vi "TEST-JSON-RPC+caraya.vi"(8 "error in (no error)":errorcluster) -> (0 "error out":errorcluster)   [LabVIEW 2019]
uses:
  TEST-JSON-RPC--Cluster.ctl
  <vilib>/numeric/Random Number (Range) DBL.vi
  <vilib>/numeric/Random Number (Range) I64.vi
  423c0946-e876-4033-917c-c4e0f5a656b4.vi
  545e0fdc-708c-4040-a6f5-a4d862a94354.vi
  85357fc9-3c23-47d6-a25c-dbb7056a88c4.vi
  9d79f0c2-35ce-467d-8164-7d449b6aa026.vi
  53d3177d-6787-4563-b3f2-ec7d47ca270a.vi
  d9266a12-4538-4804-ad7c-12d0542650b7.vi
  f59088ab-3144-40f5-84fa-71997c4bd8c3.vi
  <vilib>/numeric/sub_Random U32.vi
  <vilib>/JDP Science/JSONtext/JSON text to Variant (path).vi
  <vilib>/JDP Science/JSONtext/Find Item.vi
  <vilib>/JDP Science/JSONtext/Next JSON Value.vi
  <vilib>/JDP Science/JSONtext/String Subset.vi
  <vilib>/JDP Science/JSONtext/Parsing/Advance past next JSON Value (inlined COPY).vi
  <vilib>/JDP Science/JSONtext/Parsing/Advance past whitespace.vi
  <vilib>/JDP Science/JSONtext/Parsing/Advance past String.vi
  <vilib>/JDP Science/JSONtext/Parsing/Advance past Number.vi
  <vilib>/JDP Science/JSONtext/Parsing/Advance past Line Ending.vi
  <vilib>/JDP Science/JSONtext/JSON text to Variant.vi
  <vilib>/Utility/Data Type/Get Type Information.vi
  <vilib>/JDP Science/JSONtext/Parsing/Parse Full Path or Item Name.vi
  <vilib>/JDP Science/JSONtext/Parsing/Advance past Array.vi
  <vilib>/JDP Science/JSONtext/Parsing/Advance past Object.vi
  <vilib>/JDP Science/JSONtext/support/Error Cluster From Code.vi
  <vilib>/JDP Science/JSONtext/Offset/Find Item Locations by Path.vi
  <vilib>/addons/_JKI Toolkits/Caraya/classes/Assert/Assert Almost Equal_Float.vi
  <vilib>/JDP Science/JSONtext/LVClass Serializer/JSONtext LVClass Serializer.lvclass
  JSON-RPC/JSON-RPC.lvclass
  <vilib>/JDP Science/JSONtext/JSONtext.lvlib
  <vilib>/addons/_JKI Toolkits/Caraya/classes/Test/Test.lvclass
  <vilib>/addons/_JKI Toolkits/Caraya/classes/Assert/Assert.lvclass
  <vilib>/Utility/Data Type/NI_Data Type.lvlib
panel:
  out "Elements":dbl[](array[numeric])
  out "Names 3":string[](array[string])
  out "Params 3":string[](array[string])
  out "Array 2":dbl[][](array[numeric])
  out "Array":T1[](array[typedef])
  out "Clusters Section":dbl[](array[numeric])
  out "Arrays":dbl[][](array[numeric])
  out "Clusters":T1[](array[typedef])
  out "Params 2":string[](array[string])
  out "Names 2":string[](array[string])
  out "Params":string[](array[string])
  out "Names":string[](array[string])
  out "REQ.Methods":string
  out "Match?":bool
  out "{JSON} Response":string
  out "{JSON} Requests":string
  out "4. parse response":dbl format="%#_6p"
  out "3. create response":dbl format="%#_6p"
  out "2. parse request":dbl format="%#_6p"
  out "1. create request":dbl format="%#_6p"
  out "REQ.Params":string
  out "results":string
  in  "Numeric":i32=3
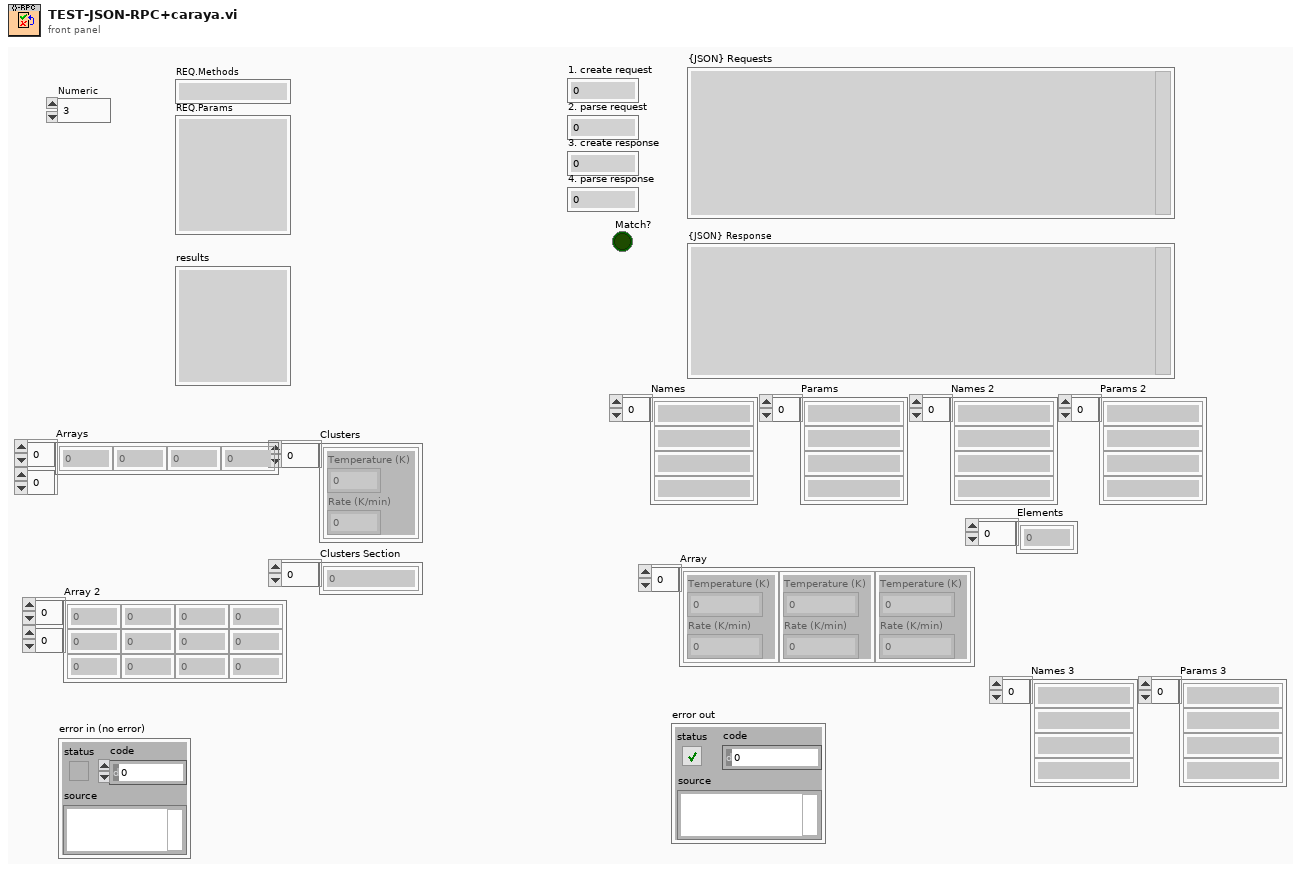
[diagram p1: front panel]
types:
  T1 = typedef "TEST-JSON-RPC--Cluster.ctl" = cluster{"Temperature (K)":dbl, "Rate (K/min)":dbl}
  T2 = enum16{"Parse Error", "Invalid Request", "Method not found", "Invalid params", "Internal error", "Server error"}
  T3 = cluster{"Temperature (K)":dbl, "Rate (K/min)":dbl}
  T4 = typedef "JSONtext.lvlib/JSON Value Type.ctl" = enum16{"Not a JSON Value", "JSON Object", "JSON Array", "String", "Number", "true", "false", "null"}
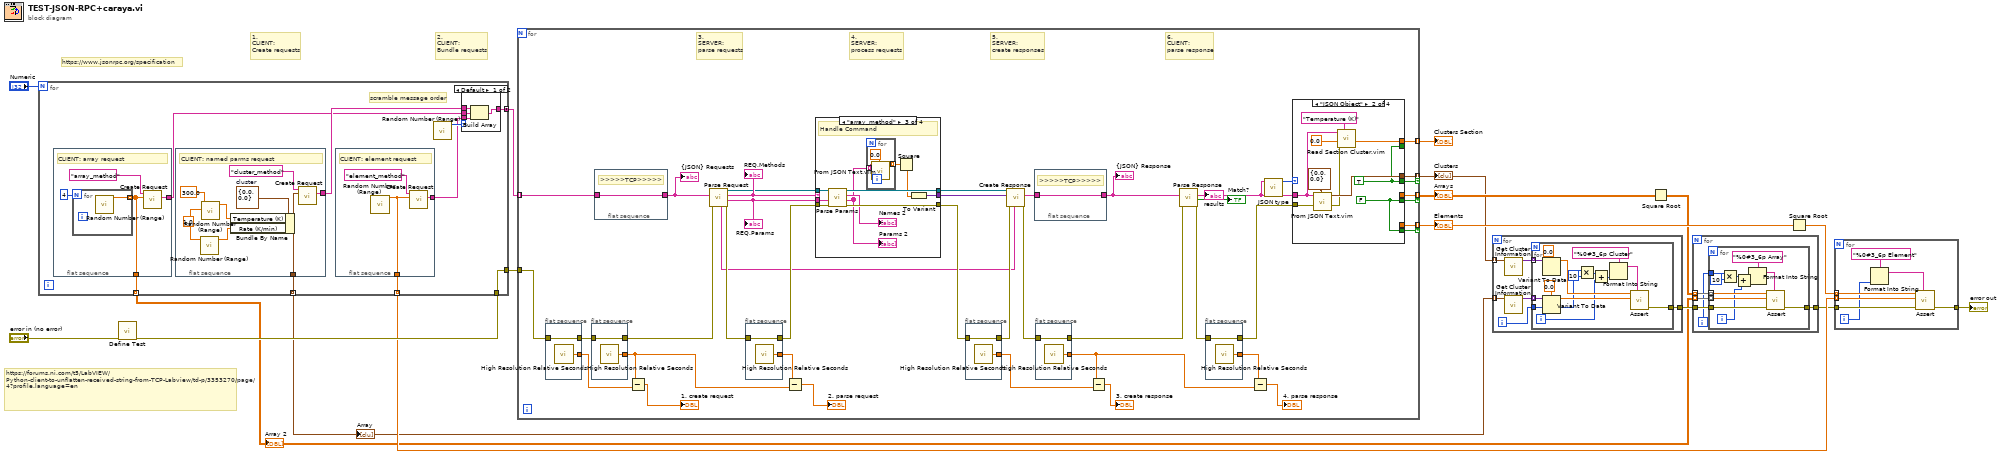
[diagram p0: block diagram]
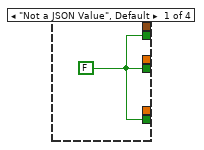
[diagram p2: hidden frame]
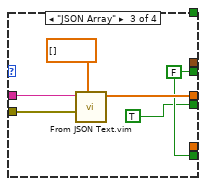
[diagram p3: hidden frame]
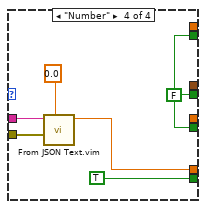
[diagram p4: hidden frame]
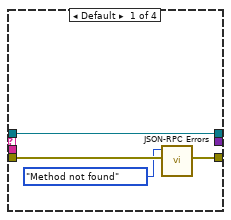
[diagram p5: hidden frame]
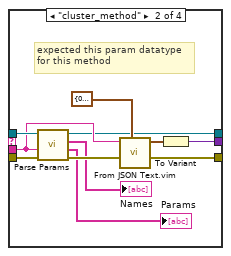
[diagram p6: hidden frame]
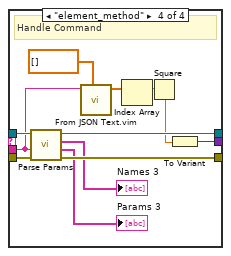
[diagram p7: hidden frame]
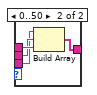
[diagram p8: hidden frame]
diagram:
  # "2.\nCLIENT:\nBundle requests"
  # "1.\nCLIENT:\nCreate requests"
  # "https://forums.ni.com/t5/LabVIEW/Python-client-to-unflatten-received-string-from-TCP-Labview/td-p/3353270/page/4?profile.language=en"
  # "https://www.jsonrpc.org/specification"
  n1 = call <vilib>:"Define Test.vi"("error in (no error)"="error in (no error)") -> ("error out"=w15:errorcluster)  [unwired: 10 in]
  n2 = for {
    N: "Numeric" -> [_]
    tunnel: [w25] -> w12 mode=concatenating
    tunnel: [w22] -> w16
    tunnel: w15 -> [w22]
    tunnel: [w21] -> w4 mode=indexing
    tunnel: [w20] -> w3 mode=indexing
    tunnel: [w18] -> w8 mode=indexing
    # "scramble message order"
    n3 = flat-sequence {
      tunnel: [w39] -> w23
      tunnel: [w38] -> w21
      frame #0 {
        # "CLIENT: array request"
        n4 = for {
          N: 4 -> [_]
          tunnel: [w42] -> w38 mode=indexing
          n5 = call-poly <vilib>:"Random Number (Range).vi"() -> ("number"=w42:dbl)  [unwired: 11 in]
        }
        n6 = call "Create Request.vi"("params"=w38, "method"="array_method" ("Request.method")) -> ("{JSON} Requests"=w39:string)  [unwired: 6 in, 3 out]
      }
    }
    n7 = flat-sequence {
      tunnel: [w33] -> w26
      tunnel: [w30] -> w20
      frame #0 {
        w35 = 1.0 ("lower bound (0)")
        w37 = T1 {"Temperature (K)"=0.0, "Rate (K/min)"=0.0}  # cluster
        # "CLIENT: named parms request"
        n8 = call-poly <vilib>:"Random Number (Range).vi"("upper bound (100)"=w35) -> ("number"=w32:dbl)  [unwired: 10 in]
        n9 = call-poly <vilib>:"Random Number (Range).vi"("lower bound (0)"=w35, "upper bound (100)"=300.0 ("lower bound (0)")) -> ("number"=w31:dbl)  [unwired: 9 in]
        n10 = Bundle By Name(cluster=w37, "Temperature (K)"=w31, "Rate (K/min)"=w32) -> (w30:T1)
        n11 = call "Create Request.vi"("params"=w30, "method"="cluster_method" ("Request.method")) -> ("{JSON} Requests"=w33:string)  [unwired: 6 in, 3 out]
      }
    }
    n12 = flat-sequence {
      tunnel: [w28] -> w19
      tunnel: [w27] -> w18
      frame #0 {
        # "CLIENT: element request"
        n13 = call-poly <vilib>:"Random Number (Range).vi"() -> ("number"=w27:dbl)  [unwired: 11 in]
        n14 = call "Create Request.vi"("params"=w27, "method"="element_method" ("Request.method")) -> ("{JSON} Requests"=w28:string)  [unwired: 6 in, 3 out]
      }
    }
    n15 = call-poly <vilib>:"Random Number (Range).vi"() -> ("number"=w24:i64)  [unwired: 11 in]
    n16 = case shown="Default" w24 {
      tunnel: w26 -> [w46 w50]
      tunnel: w23 -> [w45 w49]
      tunnel: [w44 w48] -> w25
      tunnel: w19 -> [w43 w47]
      frame Default {
        n17 = Build Array(w46, w45, w43) -> (w44:string[])
      }
      frame 0..50 {
        n18 = Build Array(w47, w49, w50) -> (w48:string[])
      }
    }
  }
  "Array" <- w3
  "Array 2" <- w4
  n19 = for {
    tunnel: w16 -> [w66]
    tunnel: [w61] -> w14 mode=indexing
    tunnel: [w60] -> w2 mode=indexing if=w51
    tunnel: [w59] -> w13 mode=indexing if=w52
    tunnel: w12 -> [w58] mode=indexing
    tunnel: [w56] -> w10 mode=indexing if=w53
    # "3.\nSERVER:\nparse requests"
    # "6.\nCLIENT:\nparse response"
    # "4.\nSERVER:\nprocess requests"
    # "5.\nSERVER:\ncreate responses"
    n20 = flat-sequence {
      tunnel: [w165] -> w57
      tunnel: [w166] -> w54
      tunnel: w66 -> [w165]
      frame #0 {
        n21 = call <vilib>:"High Resolution Relative Seconds.vi"() -> ("relative seconds"=w166:dbl)
      }
    }
    n22 = flat-sequence {
      tunnel: [w163] -> w75
      tunnel: [w164] -> w87
      tunnel: w57 -> [w163]
      frame #0 {
        n23 = call <vilib>:"High Resolution Relative Seconds.vi"() -> ("relative seconds"=w164:dbl)
      }
    }
    n24 = flat-sequence {
      tunnel: w58 -> [w168]
      tunnel: [w168] -> w73
      frame #0 {
        # ">>>>>TCP>>>>>"
      }
    }
    n25 = Subtract(x=w87, y=w54) -> (x-y=→"1. create request":dbl)
    n26 = call "Parse Request.vi"("error in (no error)"=w75, "{JSON} Request"=w73) -> ("error out"=w74:errorcluster, "Params"=w89:string, "Method"=w90:string, "JSON-RPC out"=w77:refnum<class "JSON-RPC.lvclass">, "ID"=w64:string)  [unwired: 5 in]
    "REQ.Params" <- w89
    "REQ.Methods" <- w90
    n27 = flat-sequence {
      tunnel: [w161] -> w88
      tunnel: [w162] -> w84
      tunnel: w74 -> [w161]
      frame #0 {
        n28 = call <vilib>:"High Resolution Relative Seconds.vi"() -> ("relative seconds"=w162:dbl)
      }
    }
    n29 = Subtract(x=w84, y=w87) -> (x-y=→"2. parse request":dbl)
    n30 = case shown="\"array_method\"" w90 {
      tunnel: w88 -> [w118 w124 w137 w152]
      tunnel: [w117 w129 w135 w151] -> w85
      tunnel: [_ w128 w139 w154] -> w65
      tunnel: w89 -> [_ w122 w136 w144]
      tunnel: w77 -> [w115 w123 w138 w153]
      tunnel: [w115 w121 w133 w149] -> w76
      frame Default {
        n31 = call "JSON-RPC Errors.vi"("error in"=w118, "Enum"=T2."Method not found") -> ("error out"=w117:errorcluster)  [unwired: 9 in]
      }
      frame "cluster_method" {
        # "expected this param datatype\nfor this method"
        n32 = call "Parse Params.vi"("error in (no error)"=w124, "{JSON} Params"=w122, "JSON-RPC in"=w123) -> ("error out"=w125:errorcluster, "Params"=→"Params":string[], "Names"=→"Names":string[], "JSON-RPC out"=w121:refnum<class "JSON-RPC.lvclass">)  [unwired: 5 in]
        n33 = call "From JSON Text.vim"("Data Type and Default Value"=T3 {"Temperature (K)"=0.0, "Rate (K/min)"=0.0} ("Cluster"), "error in (no error)"=w125, "JSON"=w122) -> ("error out"=w129:errorcluster, "Data out"=w126:T3)  [unwired: 7 in]
        n34 = To Variant(anything=w126) -> (Variant=w128:variant)
      }
      frame "array_method" {
        # "Handle Command"
        n35 = call "Parse Params.vi"("error in (no error)"=w137, "{JSON} Params"=w136, "JSON-RPC in"=w138) -> ("error out"=w135:errorcluster, "Params"=w132:string[], "Names"=→"Names 2":string[], "JSON-RPC out"=w133:refnum<class "JSON-RPC.lvclass">)  [unwired: 5 in]
        "Params 2" <- w132
        n36 = for {
          tunnel: w132 -> [w141] mode=indexing
          tunnel: [w140] -> w131 mode=indexing
          n37 = call "From JSON Text.vim"("Data Type and Default Value"=0.0, "JSON"=w141) -> ("Data out"=w140:dbl)  [unwired: 8 in, 1 out]
        }
        n38 = Square(x=w131) -> (x^2=w130:dbl[])
        n39 = To Variant(anything=w130) -> (Variant=w139:variant)
      }
      frame "element_method" {
        # "Handle Command"
        n40 = call "Parse Params.vi"("error in (no error)"=w152, "{JSON} Params"=w144, "JSON-RPC in"=w153) -> ("error out"=w151:errorcluster, "Params"=→"Params 3":string[], "Names"=→"Names 3":string[], "JSON-RPC out"=w149:refnum<class "JSON-RPC.lvclass">)  [unwired: 5 in]
        n41 = call "From JSON Text.vim"("Data Type and Default Value"=dbl[] [], "JSON"=w144) -> ("Data out"=w147:dbl[])  [unwired: 8 in, 1 out]
        n42 = Index Array(array=w147) -> (element=w143:dbl)  [unwired: 1 in]
        n43 = Square(x=w143) -> (x^2=w146:dbl)
        n44 = To Variant(anything=w146) -> (Variant=w154:variant)
      }
    }
    n45 = flat-sequence {
      tunnel: [w159] -> w68
      tunnel: [w160] -> w82
      tunnel: w85 -> [w159]
      frame #0 {
        n46 = call <vilib>:"High Resolution Relative Seconds.vi"() -> ("relative seconds"=w160:dbl)
      }
    }
    n47 = call "Create Response.vi"("id"=w64, "error in (no error)"=w68, "result"=w65, "JSON-RPC in"=w76) -> ("error out"=w67:errorcluster, "{JSON} Response"=w72:string)  [unwired: 5 in, 1 out]
    n48 = flat-sequence {
      tunnel: w72 -> [w167]
      tunnel: [w167] -> w69
      frame #0 {
        # ">>>>>TCP>>>>>"
      }
    }
    n49 = flat-sequence {
      tunnel: [w157] -> w71
      tunnel: [w158] -> w80
      tunnel: w67 -> [w157]
      frame #0 {
        n50 = call <vilib>:"High Resolution Relative Seconds.vi"() -> ("relative seconds"=w158:dbl)
      }
    }
    n51 = Subtract(x=w80, y=w82) -> (x-y=→"3. create response":dbl)
    n52 = call "Parse Response.vi"("error in (no error)"=w71, "{JSON} Response"=w69) -> ("error out"=w70:errorcluster, "Equal?"=→"Match?":bool, "results"=w62:string)  [unwired: 5 in, 2 out]
    "results" <- w62
    n53 = flat-sequence {
      tunnel: [w155] -> w63
      tunnel: [w156] -> w81
      tunnel: w70 -> [w155]
      frame #0 {
        n54 = call <vilib>:"High Resolution Relative Seconds.vi"() -> ("relative seconds"=w156:dbl)
      }
    }
    n55 = Subtract(x=w81, y=w80) -> (x-y=→"4. parse response":dbl)
    n56 = call <vilib>:"JSON type.vi"("JSON"=w62) -> ("JSON Value Type"=w55:T4)  [unwired: 9 in, 1 out]
    n57 = case shown="\"JSON Object\"" w55 {
      tunnel: w62 -> [_ w99 w108 w114]
      tunnel: w63 -> [_ w101 w107 w113]
      tunnel: [_ _ w105 _] -> w59
      tunnel: [w92 w93 TRUE w109] -> w52
      tunnel: [_ w100 _ _] -> w60
      tunnel: [w92 w95 w104 w109] -> w51
      tunnel: [_ w96 _ _] -> w61
      tunnel: [_ w95 _ w109] -> _
      tunnel: [_ _ _ w110] -> w56
      tunnel: [w92 w93 w104 TRUE] -> w53
      frame "Not a JSON Value", Default {
        w92 = FALSE
      }
      frame "JSON Object" {
        w95 = TRUE
        w93 = FALSE
        n58 = call "From JSON Text.vim"("Data Type and Default Value"=T1 {"Temperature (K)"=0.0, "Rate (K/min)"=0.0} ("Cluster"), "error in (no error)"=w101, "JSON"=w99) -> ("error out"=w94:errorcluster, "Data out"=w100:T1)  [unwired: 7 in]
        n59 = call "Read Section Cluster.vim"("Section (Cluster Name)"="Temperature (K)", "error in (no error)"=w94, "Section Cluster"=0.0, "JSON Sections"=w99) -> ("Cluster set from section"=w96:dbl)  [unwired: 4 in, 2 out]
      }
      frame "JSON Array" {
        w104 = FALSE
        n60 = call "From JSON Text.vim"("Data Type and Default Value"=dbl[] [], "error in (no error)"=w107, "JSON"=w108) -> ("Data out"=w105:dbl[])  [unwired: 7 in, 1 out]
      }
      frame "Number" {
        w109 = FALSE
        n61 = call "From JSON Text.vim"("Data Type and Default Value"=0.0, "error in (no error)"=w113, "JSON"=w114) -> ("Data out"=w110:dbl)  [unwired: 7 in, 1 out]
      }
    }
    "{JSON} Requests" <- w73
    "{JSON} Response" <- w69
  }
  "Clusters" <- w2
  "Arrays" <- w13
  "Clusters Section" <- w14
  "Elements" <- w10
  n62 = for {
    tunnel: w3 -> [w172] mode=indexing
    tunnel: [w174] -> w7
    tunnel: w2 -> [w173] mode=indexing
    i -> [w169]
    n63 = call <vilib>:"Get Cluster Information.vi"("variant"=w173) -> ("cluster elements"=w170:variant[])  [unwired: 9 in, 1 out]
    n64 = call <vilib>:"Get Cluster Information.vi"("variant"=w172) -> ("cluster elements"=w171:variant[])  [unwired: 9 in, 1 out]
    n65 = for {
      tunnel: [w188] -> w174
      tunnel: w171 -> [w186] mode=indexing
      tunnel: w170 -> [w187] mode=indexing
      tunnel: w169 -> [w179]
      i -> [w178]
      n66 = Variant To Data(type=0.0, Variant=w187) -> (data=w182:dbl)  [unwired: 1 in, 1 out]
      n67 = Variant To Data(type=0.0, Variant=w186) -> (data=w185:dbl)  [unwired: 1 in, 1 out]
      n68 = Multiply(x=w179, y=10) -> (x*y=w181:i32)
      n69 = Add(x=w181, y=w178) -> (x+y=w177:i32)
      n70 = Format Into String(format string="%0#3_6p Cluster" ("Label"), w177) -> (resulting string=w176:string)  [unwired: 2 in, 1 out]
      n71 = call-poly <vilib>:"Assert.vi"("Label"=w176, "Y"=w185, "X"=w182) -> ("error out"=w188:errorcluster)  [unwired: 8 in]
    }
  }
  n72 = Square Root(x=w13) -> (sqrt(x)=w1:dbl[][])
  n73 = for {
    tunnel: w4 -> [w193] mode=indexing
    tunnel: w1 -> [w192] mode=indexing
    tunnel: [w191] -> w5
    tunnel: w7 -> [w190]
    i -> [w189]
    n74 = for {
      tunnel: w193 -> [w204] mode=indexing
      tunnel: w192 -> [w203] mode=indexing
      tunnel: [w202] -> w191
      tunnel: w190 -> [w201]
      tunnel: w189 -> [w198]
      i -> [w195]
      n75 = Multiply(x=w198, y=10) -> (x*y=w196:i32)
      n76 = Add(x=w196, y=w195) -> (x+y=w194:i32)
      n77 = Format Into String(format string="%0#3_6p Array" ("Label"), w194) -> (resulting string=w199:string)  [unwired: 2 in, 1 out]
      n78 = call-poly <vilib>:"Assert.vi"("Label"=w199, "error in (no error)"=w201, "Y"=w204, "X"=w203) -> ("error out"=w202:errorcluster)  [unwired: 7 in]
    }
  }
  n79 = Square Root(x=w10) -> (sqrt(x)=w9:dbl[])
  n80 = for {
    tunnel: w8 -> [w211] mode=indexing
    tunnel: w9 -> [w210] mode=indexing
    tunnel: [w209] -> w6
    tunnel: w5 -> [w208]
    i -> [w207]
    n81 = Format Into String(format string="%0#3_6p Element" ("Label"), w207) -> (resulting string=w205:string)  [unwired: 2 in, 1 out]
    n82 = call-poly <vilib>:"Assert.vi"("Label"=w205, "error in (no error)"=w208, "Y"=w211, "X"=w210) -> ("error out"=w209:errorcluster)  [unwired: 7 in]
  }
  "error out" <- w6
